vi "Test API Execution from Invalid Project Path.vi"(8 "error in (no error)":errorcluster, 11 "API Test in":refnum<class "API Test.lvclass">) -> (0 "error out":errorcluster, 3 "API Test out":refnum<class "API Test.lvclass">)   [LabVIEW 2020, in "LUnit Tests.lvlib" / "API Test.lvclass"]
uses:
  API Test.lvclass
  C:/Program Files (x86)/National Instruments/LabVIEW 2020/vi.lib/Astemes/LUnit/Test Case.lvclass
  <vilib>/Astemes/LUnit/Test Case.lvclass/Test Case.ctl
  <vilib>/Astemes/LUnit/LUnit Assertion Result.lvclass/LUnit Assertion Result.ctl
  <vilib>/Astemes/LUnit/LUnit Test Case Result.lvclass/LUnit Test Case Result.ctl
  <vilib>/Astemes/LUnit/LUnit Method Result.lvclass/LUnit Method Result.ctl
  <vilib>/Astemes/LUnit/Palette/Fail.vi
  <vilib>/Astemes/LUnit/Palette/Pass.vi
  <vilib>/Astemes/LUnit/Set Assertion Type.vi
  <vilib>/Astemes/LUnit/Add test result.vi
  <vilib>/Astemes/LUnit/LUnit Write Passed.vi
  <vilib>/Astemes/LUnit/LUnit Write Message.vi
  <vilib>/Astemes/LUnit/LUnit Write Description.vi
  <vilib>/Astemes/LUnit/LUnit Write Assertion Type.vi
  <vilib>/Astemes/LUnit/LUnit Record Assertion Result.vi
  <vilib>/Astemes/LUnit/LUnit Aggregate Assertion Results.vi
  <vilib>/Astemes/LUnit/Assertion Result/LUnit Read Status.vi
  <vilib>/Astemes/LUnit/LUnit Read Message.vi
  <vilib>/Astemes/LUnit/LUnit Read Description.vi
  <vilib>/Astemes/LUnit/Method Result/LUnit Merge Status.vi
  <vilib>/Astemes/LUnit/LUnit Concatenate result strings.vi
  <vilib>/Astemes/LUnit/LUnit Assertion Result.lvclass
  API Test.lvclass/API Test.ctl
  source/Framework/Execution API/Execution API.lvclass
  <vilib>/Astemes/LUnit/Test Case.lvclass
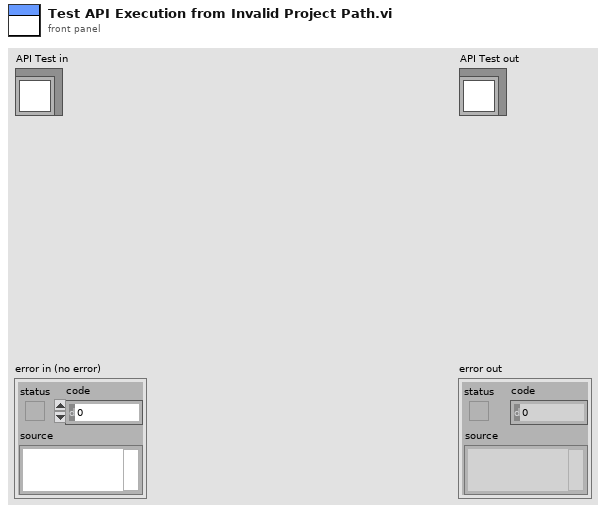
[diagram p1: front panel]
types:
  T1 = cluster{"Event Registration Refnum":refnum<event-registration>, "Event Registration Refnum":refnum<event-registration>}
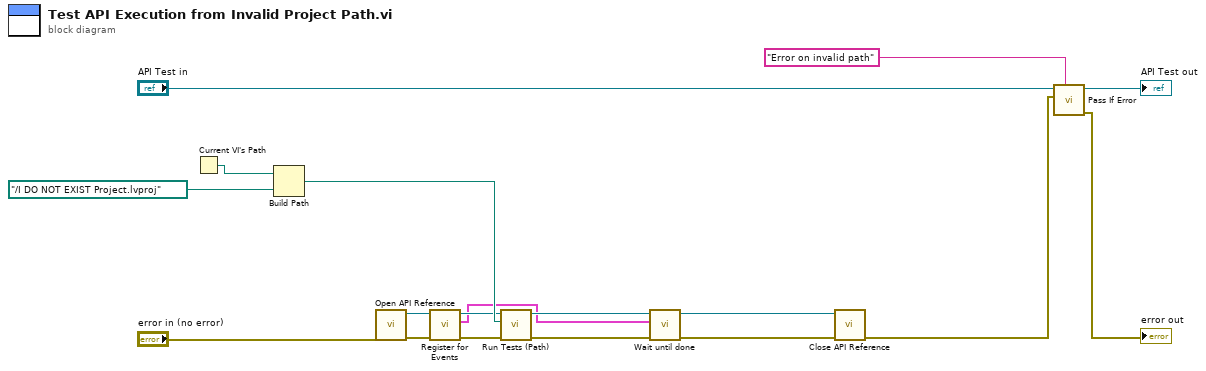
[diagram p0: block diagram]
diagram:
  n1 = Current VI's Path() -> (path=w12:path)
  n2 = Build Path(base path=w12, name or relative path=path "../I DO NOT EXIST Project.lvproj" ("class path")) -> (appended path=w10:path)
  n3 = call "Open API Reference.vi"("error in (no error)"="error in (no error)") -> ("error out"=w8:errorcluster, "Execution API out"=w9:refnum<class "Execution API.lvclass">)  [unwired: 9 in]
  n4 = call "Register for Events.vi"("error in (no error)"=w8, "Execution API In"=w9) -> ("error out"=w7:errorcluster, "Result Events Registration"=w1:T1, "Execution API Out"=w6:refnum<class "Execution API.lvclass">)  [unwired: 7 in]
  n5 = call "Run Tests (Path).vi"("error in (no error)"=w7, "Project or Class Path"=w10, "Execution API In"=w6) -> ("error out"=w3:errorcluster, "Execution API Out"=w5:refnum<class "Execution API.lvclass">)  [unwired: 7 in]
  n6 = call "Wait until done.vi"("error in (no error)"=w3, "Result Events"=w1, "Execution API In"=w5) -> ("error out"=w2:errorcluster, "Execution API Out"=w4:refnum<class "Execution API.lvclass">)  [unwired: 6 in, 1 out]
  n7 = call "Close API Reference.vi"("error in (no error)"=w2, "Execution API in"=w4) -> ("error out"=w16:errorcluster)  [unwired: 9 in]
  n8 = call <vilib>:"Pass If Error.vi"("Description"="Error on invalid path", "Assert error"=w16, "LUnit Test Case In"="API Test in") -> ("error out"=→"error out":errorcluster, "LUnit Test Case Out"=→"API Test out":refnum<class "API Test.lvclass">)  [unwired: 7 in]
